vi "Main.vi"() -> (0 "error out":errorcluster)   [LabVIEW 2020, in "Program.lvclass"]
uses:
  Program.lvclass
  ProxyImage_class/ProxyImage.lvclass
  Console_class/Console.lvclass
panel:
  out "TextOut":string
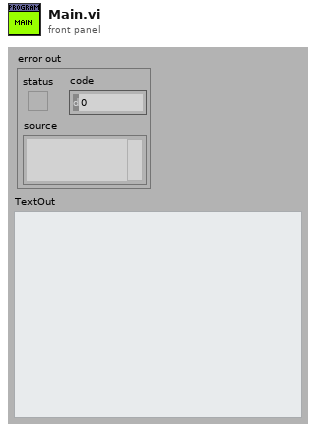
[diagram p1: front panel]
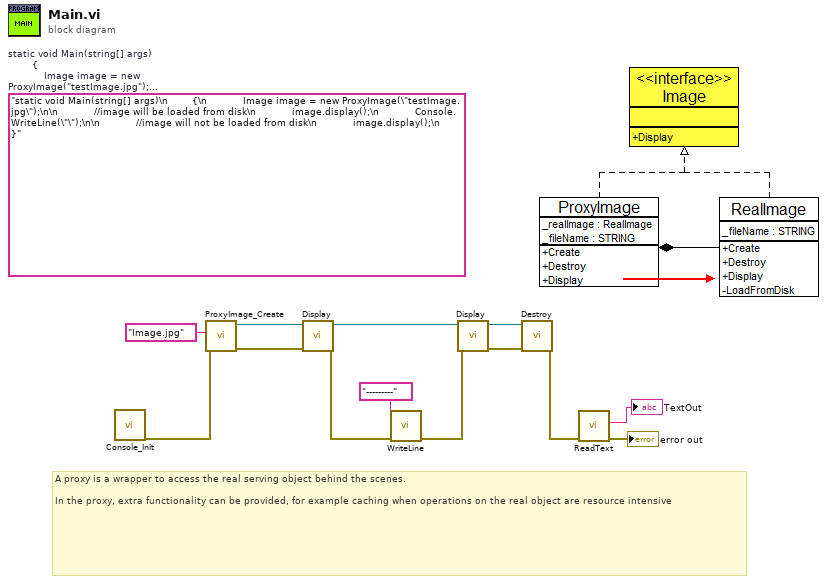
[diagram p0: block diagram]
diagram:
  (unwired) "static void Main(string[] args)\n        {\n            Image image = new ProxyImage(\"testImage.jpg\");\n\n            //image will be loaded from disk\n            image.display();\n            Console.WriteLine(\"\");\n\n            //image will not be loaded from disk\n            image.display();\n        }"  # static void Main(string[] args)         {             Image image = new ProxyImage("testImage.jpg");              //image will be loaded from disk             image.display();             Console.WriteLine("");              //image will not be loaded from disk             image.display();         }
  # "A proxy is a wrapper to access the real serving object behind the scenes.\n\nIn the proxy, extra functionality can be provided, for example caching when operations on the real object are resource intensive"
  n1 = call "Console_Init.vi"() -> ("Error Out"=w10:errorcluster)  [unwired: 10 in, 1 out]
  n2 = call "ProxyImage_Create.vi"("Error In"=w10, "FileName"="Image.jpg") -> ("Error Out"=w9:errorcluster, "reference out"=w12:refnum<class "ProxyImage.lvclass">)  [unwired: 8 in]
  n3 = call-dynamic "Display.vi"("Error In"=w9, "reference in"=w12) -> ("Error Out"=w7:errorcluster, "reference out"=w11:refnum<class "ProxyImage.lvclass">)  [unwired: 8 in]
  n4 = call "WriteLine.vi"("Error In"=w7, "ConsoleText"="---------") -> ("Error Out"=w6:errorcluster)  [unwired: 9 in]
  n5 = call-dynamic "Display.vi"("Error In"=w6, "reference in"=w11) -> ("Error Out"=w4:errorcluster, "reference out"=w5:refnum<class "ProxyImage.lvclass">)  [unwired: 8 in]
  n6 = call-dynamic "Destroy.vi"("Error In"=w4, "reference in"=w5) -> ("Error Out"=w3:errorcluster)  [unwired: 8 in, 1 out]
  n7 = call "ReadText.vi"("Error In"=w3) -> ("Error Out"=→"error out":errorcluster, "TextOut"=→"TextOut":string)  [unwired: 9 in]
